vi "checkFirstTimestamp.vi"(8 "error in (no error)":errorcluster, 11 "TrapezoidalWave in":refnum<class "TrapezoidalWave.lvclass">) -> (0 "error out":errorcluster, 2 "IsFirst":bool, 3 "TrapezoidalWave out":refnum<class "TrapezoidalWave.lvclass">)   [LabVIEW 2015, in "TrapezoidalWave.lvclass"]
uses:
  TrapezoidalWave.lvclass
  TrapezoidalWave.lvclass/TrapezoidalWave.ctl
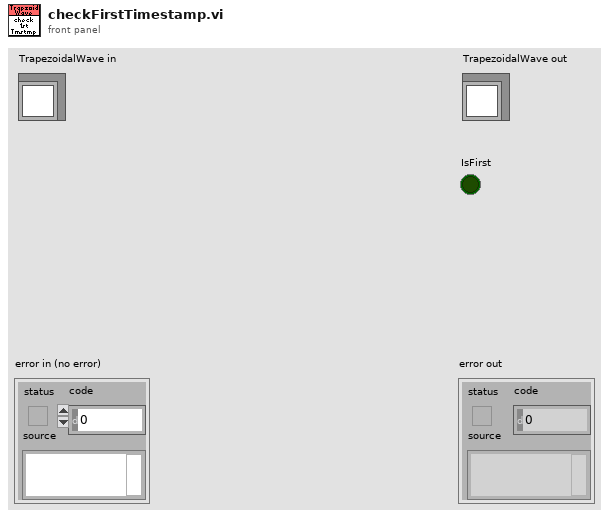
[diagram p1: front panel]
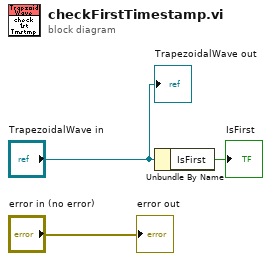
[diagram p0: block diagram]
diagram:
  n1 = Unbundle By Name("TrapezoidalWave in") -> ("IsFirst"=→"IsFirst":bool)
  "error out" <- "error in (no error)"
  "TrapezoidalWave out" <- "TrapezoidalWave in"
